vi "threhsold IMAQ.vi"(8 "error in (no error)":errorcluster, 10 "Threshold":dbl, 11 "Refnum in":T1) -> (0 "error out":errorcluster, 1 "Maximal Value":sgl, 2 "Mean Value":sgl, 3 "Refnum out":T1(plugin-control))   [LabVIEW 2020]
uses:
  IMAQ Image.ctl
  NI_Vision_Development_Module.lvlib
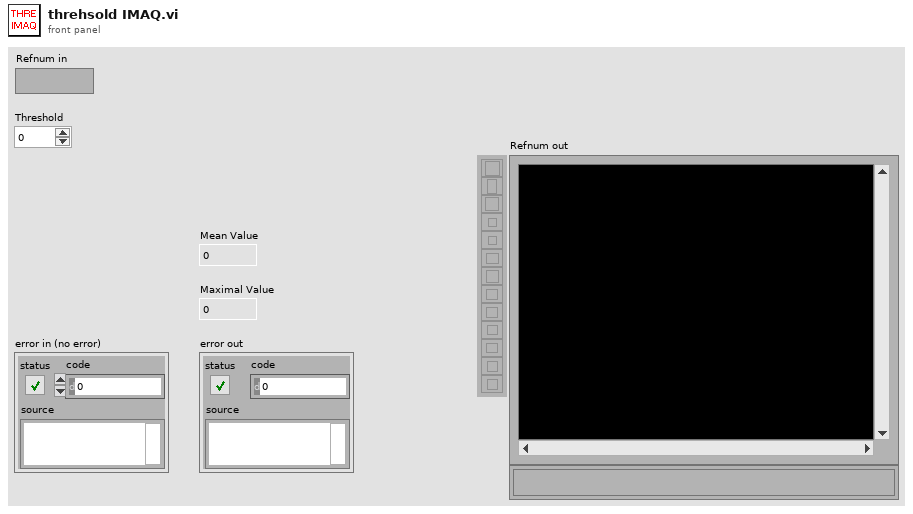
[diagram p1: front panel]
types:
  T1 = typedef "IMAQ Image.ctl" = refnum<image>
  T2 = cluster{"histogram":u32[], "Minimal Value":sgl, "Maximal Value":sgl, "Starting Value":sgl, "Interval Width":sgl, "Mean Value":sgl, "Standard  Variation":sgl, "Area (pixels)":i32}
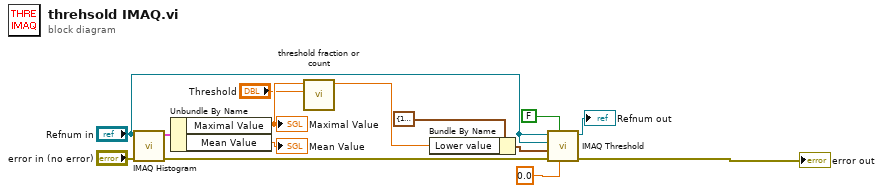
[diagram p0: block diagram]
diagram:
  n1 = call "IMAQ Histogram"("error in (no error)"="error in (no error)", "Image"="Refnum in") -> ("error out"=w7:errorcluster, "Histogram Report"=w2:T2)  [unwired: 8 in]
  n2 = Unbundle By Name(w2) -> ("Maximal Value"=w13:sgl, "Mean Value"=→"Mean Value":sgl)
  "Maximal Value" <- w13
  n3 = call "threshold fraction or count.vi"("Threshold in"="Threshold", "Maximal Value"=w13) -> ("Threshold out"=w8:dbl)  [unwired: 9 in]
  n4 = Bundle By Name(cluster=cluster{"Lower value":sgl, "Upper value":sgl} {"Lower value"=100.0, "Upper value"=9999999.0} ("Range"), "Lower value"=w8) -> (w3:cluster{"Lower value":sgl, "Upper value":sgl})
  n5 = call "IMAQ Threshold"("Replace Value"=sgl 0.0, "Keep/Replace Value (Replace)"=FALSE, "error in (no error)"=w7, "Range"=w3, "Image Dst"="Refnum in", "Image Src"="Refnum in") -> ("error out"=→"error out":errorcluster, "Image Dst Out"=→"Refnum out":T1)  [unwired: 4 in]
